vi "Receive Message Queue.vi"(8 "error in (no error)":errorcluster) -> (0 "error out":errorcluster, 3 "queue out":refnum<queue>)   [LabVIEW 2010, in "Visualizer.lvlib"]
uses:
  Visualizer.lvlib
  Message.ctl
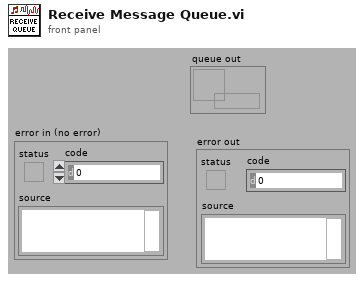
[diagram p1: front panel]
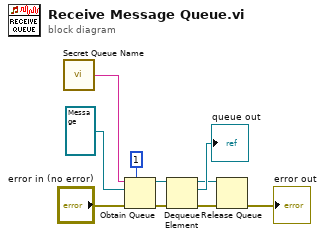
[diagram p0: block diagram]
diagram:
  n1 = call "Secret Queue Name.vi"() -> ("name (unnamed)"=w2:string)
  n2 = Obtain Queue(max queue size (-1, unlimited)=1, name (unnamed)=w2, element data type=refnum<queue> refnum ("queue out"), error in (no error)="error in (no error)") -> (queue out=w6:refnum<queue>, error out=w5:errorcluster)  [unwired: 1 in, 1 out]
  n3 = Dequeue Element(queue=w6, error in (no error)=w5) -> (queue out=w8:refnum<queue>, element=→"queue out":refnum<queue>, error out=w7:errorcluster)  [unwired: 1 in, 1 out]
  n4 = Release Queue(queue=w8, error in (no error)=w7) -> (error out=→"error out":errorcluster)  [unwired: 1 in, 2 out]
